vi "Start CAN Task.vi"(8 "error in":errorcluster, 11 "CANopen Master in":refnum<class "CANopen Master.lvclass">) -> (0 "error out":errorcluster, 3 "CANopen Master out":refnum<class "CANopen Master.lvclass">)   [LabVIEW 2024, in "CANopen Master.lvlib" / "CANopen Master.lvclass"]
uses:
  CANopen Master.lvclass
  CANopen Master.lvclass/CANopen Master.ctl
  CAN Task.vi
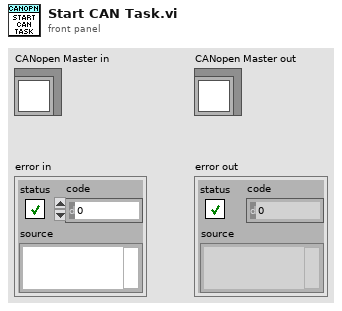
[diagram p1: front panel]
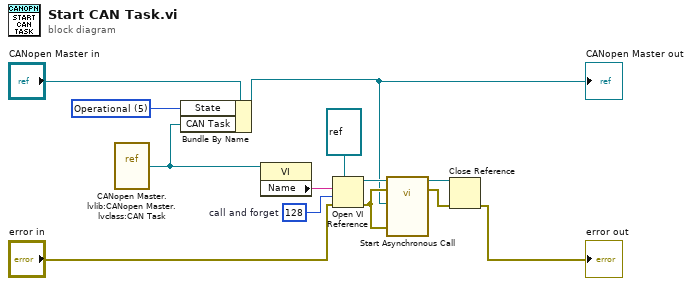
[diagram p0: block diagram]
diagram:
  w5 = u16 5 items=["Boot-Up"=0, "Stopped"=4, "Operational"=5, "Pre-Operational"=127] ("State")
  w12 = 128  # call and forget
  n1 = vi-ref "CANopen Master.lvlib:CANopen Master.lvclass:CAN Task.vi"() -> (w1:refnum<vi>)
  n2 = Bundle By Name(cluster="CANopen Master in", "State"=w5, "CAN Task"=w1) -> (w3:refnum<class "CANopen Master.lvclass">)
  "CANopen Master out" <- w3
  n3 = property class="VI"(reference=w1) -> ("Name"=w6:string)  [unwired: 1 in, 2 out]
  n4 = Open VI Reference(type specifier VI Refnum (for type only)=refnum<vi> refnum, vi path=w6, options=w12, error in (no error)="error in") -> (vi reference=w11:refnum<vi>, error out=w7:errorcluster)  [unwired: 2 in]
  n5 = call-by-ref "Start Asynchronous Call"(reference=w11, error in=w7, "error in"=w7, "CANopen Master in"=w3) -> (reference out=w2:refnum<vi>, error out=w10:errorcluster)  [unwired: 10 in]
  n6 = Close Reference(reference=w2, error in (no error)=w10) -> (error out=→"error out":errorcluster)
